vi "Arret_Urgence_Handler.vi"(8 "Error In":errorcluster caption="Entrée d'erreur", 11 "Donnees_Globales_IN":T1) -> (0 "Error Out":errorcluster caption="Sortie d'erreur", 3 "Donnees_Globale_Out":T1)   [LabVIEW 2019]
uses:
  Asc_State_Inputs.ctl
  Etat_Asc.ctl
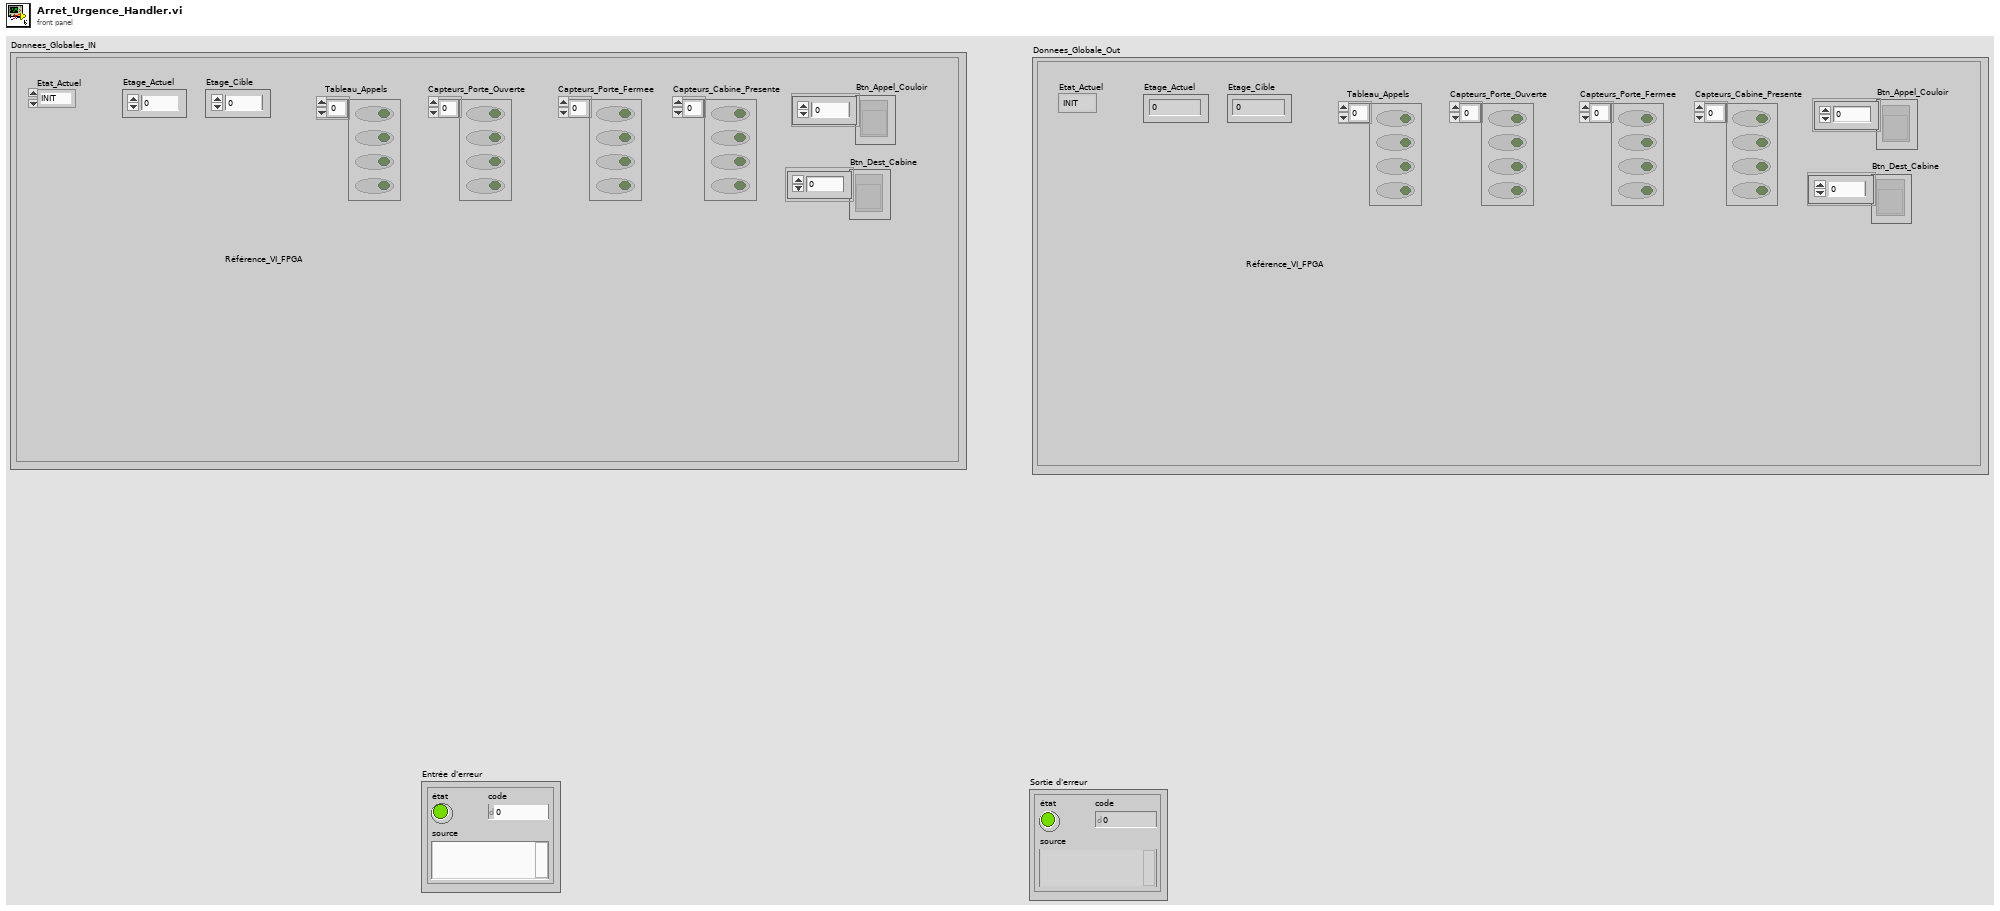
[diagram p1: front panel]
types:
  T1 = typedef "Asc_State_Inputs.ctl" = cluster{"Etage_Actuel":i32, "Etat_Actuel":T2, "Etage_Cible":i32, "Tableau_Appels":bool[], "Capteurs_Porte_Ouverte":bool[], "Capteurs_Porte_Fermee":bool[], "Capteurs_Cabine_Presente":bool[], "Btn_Appel_Couloir":refnum<vi>[], "Btn_Dest_Cabine":refnum<vi>[], "Référence_VI_FPGA":refnum<k20>}
  T2 = typedef "Etat_Asc.ctl" = enum16{"INIT", "REPOS", "DEPLACEMENT", "OUVERTURE_PORTE", "ATTENTE_TEMPO", "FERMETURE_PORTE", "ARRET_URGENCE"}
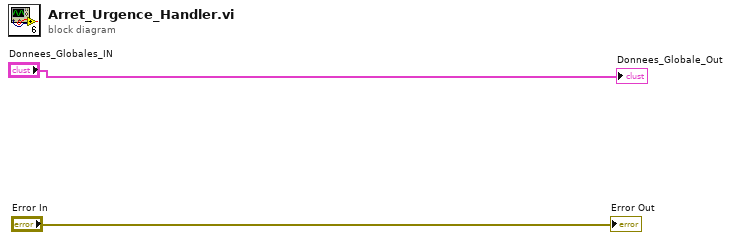
[diagram p0: block diagram]
diagram:
  "Donnees_Globale_Out" <- "Donnees_Globales_IN"
  "Error Out" <- "Error In"
